vi "Check position range.vi"(8 "error in (no error)":errorcluster, 10 "motor position":string, 11 "Motor in":refnum<class "Motor.lvclass">) -> (0 "error out":errorcluster, 1 "modified":bool, 2 "in-range position":string, 3 "Motor out":refnum<class "Motor.lvclass">)   [LabVIEW 2018, in "Motor.lvclass"]
uses:
  Motor.lvclass
  Motor.lvclass/Motor.ctl
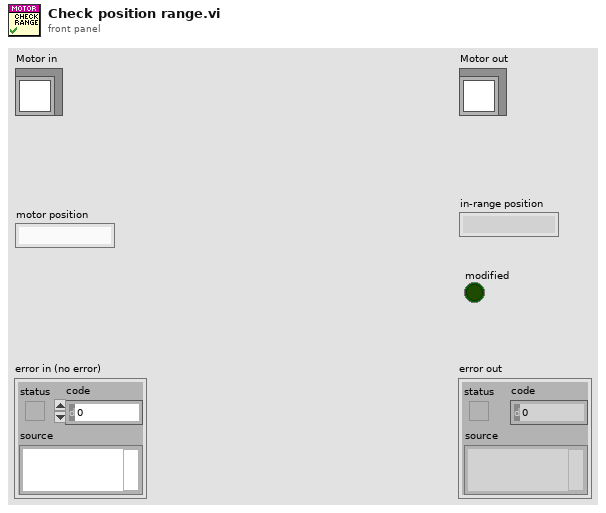
[diagram p1: front panel]
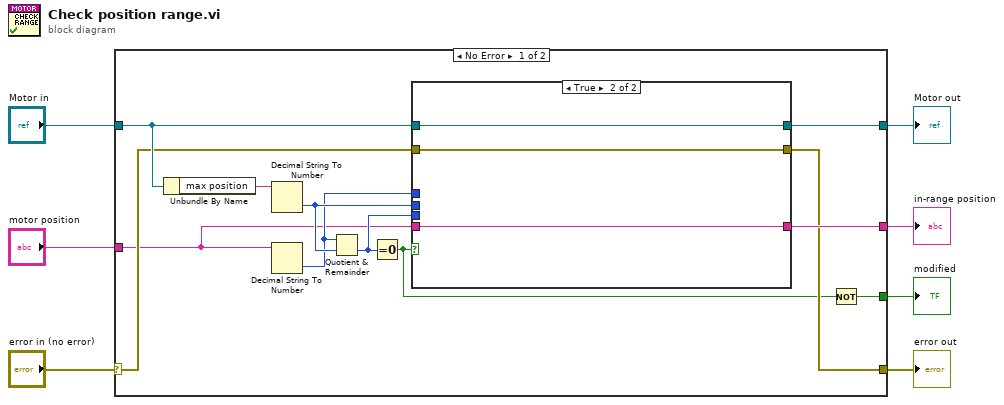
[diagram p0: block diagram]
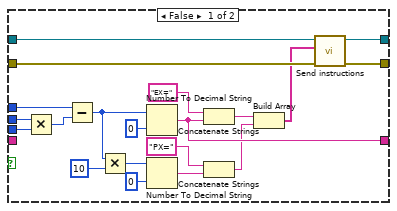
[diagram p2: hidden frame]
diagram:
  n1 = case shown="No Error" "error in (no error)" {
    selector: "error in (no error)" -> [w12 w43]
    tunnel: [w11 w43] -> w6
    tunnel: [w13 w44] -> w4
    tunnel: "Motor in" -> [w14 w44]
    tunnel: "motor position" -> [w8 _]
    tunnel: [w15 _] -> w2
    tunnel: [w9 _] -> w1
    frame No Error {
      n2 = Unbundle By Name(w14) -> ("max position"=w19:string)
      n3 = Decimal String To Number(string=w19) -> (number=w17:i32)  [unwired: 2 in, 1 out]
      n4 = Decimal String To Number(string=w8) -> (number=w16:i32)  [unwired: 2 in, 1 out]
      n5 = Quotient & Remainder(x=w16, y=w17) -> (floor(x/y)=w18:i32)  [unwired: 1 out]
      n6 = Equal To 0?(x=w18) -> (x = 0?=w10:bool)
      n7 = case shown="True" w10 {
        tunnel: w18 -> [w39 _]
        tunnel: w17 -> [w37 _]
        tunnel: w16 -> [w36 _]
        tunnel: [w27 w40] -> w15
        tunnel: w14 -> [w24 w42]
        tunnel: [w23 w42] -> w13
        tunnel: w12 -> [w22 w41]
        tunnel: [w21 w41] -> w11
        tunnel: w8 -> [_ w40]
        frame False {
          n8 = Multiply(x=w37, y=w39) -> (x*y=w38:i32)
          n9 = Subtract(x=w36, y=w38) -> (x-y=w32:i32)
          n10 = Multiply(x=w32, y=10) -> (x*y=w33:i32)
          n11 = Number To Decimal String(number=w32, width (-)=i16 0) -> (decimal integer string=w27:string)
          n12 = Number To Decimal String(number=w33, width (-)=i16 0) -> (decimal integer string=w30:string)
          n13 = Concatenate Strings("EX=" ("string"), w27) -> (w26:string)
          n14 = Concatenate Strings("PX=" ("string"), w30) -> (w25:string)
          n15 = Build Array(w26, w25) -> (w20:string[])
          n16 = call-dynamic "Send instructions.vi"("error in (no error)"=w22, "instructions"=w20, "Motor in"=w24) -> ("error out"=w21:errorcluster, "Motor out"=w23:refnum<class "Motor.lvclass">)  [unwired: 4 in, 3 out]
        }
        frame True {
        }
      }
      n17 = Not(x=w10) -> (.not. x?=w9:bool)
    }
    frame Error {
    }
  }
  "error out" <- w6
  "Motor out" <- w4
  "in-range position" <- w2
  "modified" <- w1
